vi "Validate Discrete Input Mapping.vi"(8 "error in (no error)":errorcluster, 10 "Mapping":u16) -> (0 "error out":errorcluster, 1 "Status Message":string, 3 "Valid?":bool)   [LabVIEW 2015]
uses:
  Modbus Master System Explorer.lvlib
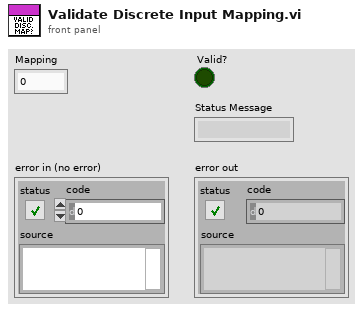
[diagram p1: front panel]
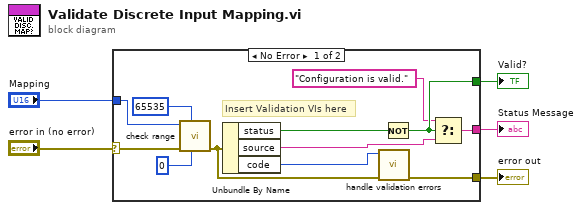
[diagram p0: block diagram]
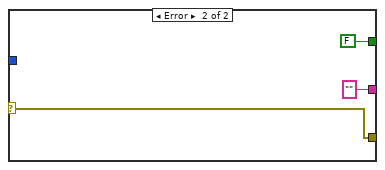
[diagram p2: hidden frame]
diagram:
  n1 = case shown="No Error" "error in (no error)" {
    selector: "error in (no error)" -> [w12 w20]
    tunnel: "Mapping" -> [w11 _]
    tunnel: [w6 w20] -> w3
    tunnel: [w16 FALSE] -> w2
    tunnel: [w13 "" ("source")] -> w1
    frame No Error {
      # "Insert Validation VIs here"
      n2 = call "check range.vi"("lower limit"=0, "upper limit"=65535, "error in (no error)"=w12, "Mapping"=w11) -> ("error out"=w7:errorcluster)  [unwired: 7 in]
      n3 = Unbundle By Name(w7) -> ("status"=w17:bool, "source"=w14:string, "code"=w8:i32)
      n4 = call "handle validation errors.vi"("error in (no error)"=w7, "code"=w8) -> ("error out"=w6:errorcluster)  [unwired: 9 in]
      n5 = Not(x=w17) -> (.not. x?=w16:bool)
      n6 = Select(t="Configuration is valid." ("source"), s=w16, f=w14) -> (s? t:f=w13:string)
    }
    frame Error {
    }
  }
  "error out" <- w3
  "Valid?" <- w2
  "Status Message" <- w1
